vi "SetWaitFor_popup.vi"(0 "Input Line Command":string, 3 "error in (no error)":errorcluster) -> (8 "error out":errorcluster, 9 "Cancel":bool, 10 "Output Line Command":string)   [LabVIEW 2020]
panel:
  in  "platform":u16(ring) items=["Mac", "PC"]
  in  "Cancel button":bool
  in  "OK Button":bool
  in  "Unit":string(combo)="s"
  in  "Wait for":string
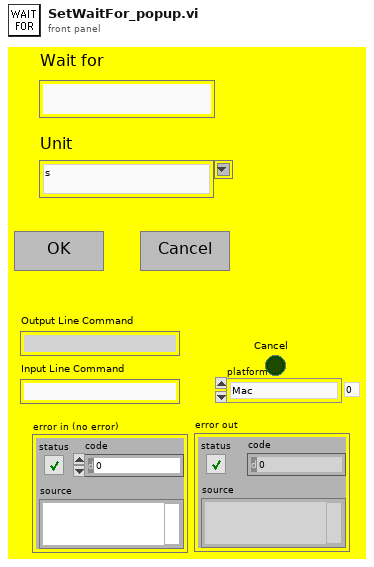
[diagram p1: front panel]
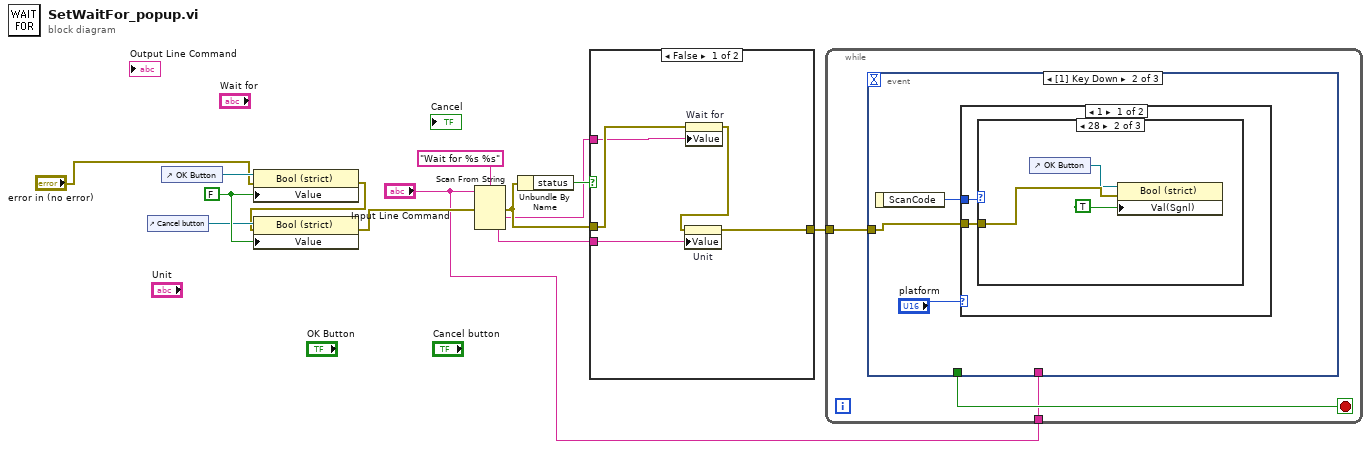
[diagram p0: block diagram]
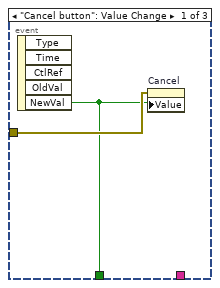
[diagram p2: hidden frame]
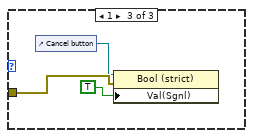
[diagram p4: hidden frame]
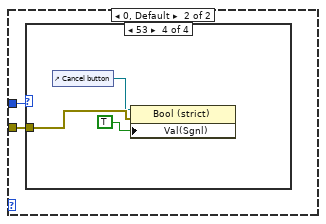
[diagram p5: hidden frame]
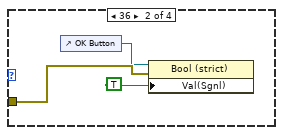
[diagram p7: hidden frame]
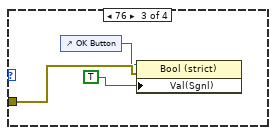
[diagram p8: hidden frame]
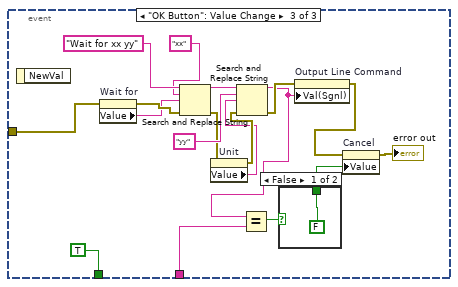
[diagram p9: hidden frame]
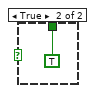
[diagram p10: hidden frame]
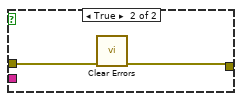
[diagram p11: hidden frame]
diagram:
  w13 = FALSE
  n1 = control-ref of="Cancel button"() -> (w11:refnum<vi>)
  n2 = control-ref of="OK Button"() -> (w12:refnum<vi>)
  n3 = property on="Property Node" class="Bool (strict)"(reference=w12, error in="error in (no error)", "Value"=w13) -> (error out=w9:errorcluster)  [unwired: 1 out]
  n4 = property on="Property Node" class="Bool (strict)"(reference=w11, error in=w9, "Value"=w13) -> (error out=w8:errorcluster)  [unwired: 1 out]
  n5 = Scan From String(format string="Wait for %s %s", input string="Input Line Command", error in=w8) -> (error out=w5:errorcluster, output 1=w4:string, output 2=w3:string)  [unwired: 3 in, 2 out]
  n6 = Unbundle By Name(w5) -> ("status"=w6:bool)
  n7 = case shown="False" w6 {
    tunnel: w5 -> [w18 w20]
    tunnel: w4 -> [w14 _]
    tunnel: w3 -> [w16 _]
    tunnel: [w15 w19] -> w2
    frame False {
      n8 = property on="Wait for" class="Str"(error in=w18, "Value"=w14) -> (error out=w17:errorcluster)  [unwired: 1 in, 1 out]
      n9 = property on="Unit" class="CmbBox"(error in=w17, "Value"=w16) -> (error out=w15:errorcluster)  [unwired: 1 in, 1 out]
    }
    frame True {
      n10 = call <vilib>:"Clear Errors.vi"("error in (no error)"=w20) -> ("error out"=w19:errorcluster)  [unwired: 5 in, 1 out]
    }
  }
  n11 = while {
    tunnel: w2 -> [w23]
    tunnel: "Input Line Command" -> [w21]
    stop <- w22 stop-if-true
    n12 = event shown="[1] Key Down" {
      selector: _ -> [_ _ _]
      dyn-events: _ -> [_ _ _]
      timeout: _ -> [_ _ _]
      tunnel: w23 -> [w25 w27 w62]
      tunnel: [w24 _ TRUE] -> w22
      tunnel: w21 -> [_ _ w48]
      event "Cancel button": Value Change {
        n13 = event-data() -> ("NewVal"=w24:bool)  [unwired: 1 in, 4 out]
        n14 = property on="Cancel" class="Bool (strict)"(error in=w25, "Value"=w24) -> ()  [unwired: 1 in, 2 out]
      }
      event Key Down {
        n15 = event-data() -> ("ScanCode"=w28:i16)  [unwired: 1 in]
        n16 = case shown="1" "platform" {
          tunnel: w28 -> [w30 w38]
          tunnel: w27 -> [w29 w37]
          frame 1 {
            n17 = case shown="28" w30 {
              tunnel: w29 -> [_ w33 w35]
              frame Default {
              }
              frame 28 {
                n18 = control-ref of="OK Button"() -> (w31:refnum<vi>)
                n19 = property on="Property Node" class="Bool (strict)"(reference=w31, error in=w33, "Val(Sgnl)"=TRUE ("Value (Signaling)")) -> ()  [unwired: 2 out]
              }
              frame 1 {
                n20 = control-ref of="Cancel button"() -> (w34:refnum<vi>)
                n21 = property on="Property Node" class="Bool (strict)"(reference=w34, error in=w35, "Val(Sgnl)"=TRUE ("Value (Signaling)")) -> ()  [unwired: 2 out]
              }
            }
          }
          frame 0, Default {
            n22 = case shown="53" w38 {
              tunnel: w37 -> [_ w41 w44 w46]
              frame Default {
              }
              frame 36 {
                n23 = control-ref of="OK Button"() -> (w39:refnum<vi>)
                n24 = property on="Property Node" class="Bool (strict)"(reference=w39, error in=w41, "Val(Sgnl)"=TRUE ("Value (Signaling)")) -> ()  [unwired: 2 out]
              }
              frame 76 {
                n25 = control-ref of="OK Button"() -> (w42:refnum<vi>)
                n26 = property on="Property Node" class="Bool (strict)"(reference=w42, error in=w44, "Val(Sgnl)"=TRUE ("Value (Signaling)")) -> ()  [unwired: 2 out]
              }
              frame 53 {
                n27 = control-ref of="Cancel button"() -> (w45:refnum<vi>)
                n28 = property on="Property Node" class="Bool (strict)"(reference=w45, error in=w46, "Val(Sgnl)"=TRUE ("Value (Signaling)")) -> ()  [unwired: 2 out]
              }
            }
          }
        }
      }
      event "OK Button": Value Change {
        n29 = event-data() -> ()  [unwired: 1 in, 1 out]
        n30 = property on="Wait for" class="Str"(error in=w62) -> (error out=w61:errorcluster, "Value"=w52:string)  [unwired: 1 in, 1 out]
        n31 = Search and Replace String(input string="Wait for xx yy" ("format string"), search string="xx", replace string=w52, error in=w61) -> (result string=w60:string, error out=w57:errorcluster)  [unwired: 4 in, 2 out]
        n32 = property on="Unit" class="CmbBox"(error in=w57) -> (error out=w56:errorcluster, "Value"=w55:string)  [unwired: 1 in, 1 out]
        n33 = Search and Replace String(input string=w60, search string="yy", replace string=w55, error in=w56) -> (result string=w49:string, error out=w58:errorcluster)  [unwired: 4 in, 2 out]
        n34 = Equal?(x=w49, y=w48) -> (x = y?=w51:bool)
        n35 = case shown="False" w51 {
          tunnel: [FALSE ("Cancel") TRUE ("Cancel")] -> w50
          frame False {
          }
          frame True {
          }
        }
        n36 = property on="Output Line Command" class="Str"(error in=w58, "Val(Sgnl)"=w49) -> (error out=w54:errorcluster)  [unwired: 1 in, 1 out]
        n37 = property on="Cancel" class="Bool (strict)"(error in=w54, "Value"=w50) -> (error out=→"error out":errorcluster)  [unwired: 1 in, 1 out]
      }
    }
  }
